vi "returns remaining heater time delay subvi$.vi"(0 "VISA resource name 2":refnum<visa-resource-name>="GPIB0::12::INSTR", 1 "error in (no error) 2":errorcluster) -> (2 "VISA resource name out 2":refnum<visa-resource-name>, 3 "result string":string, 4 "error out 2":errorcluster)   [LabVIEW 2009]
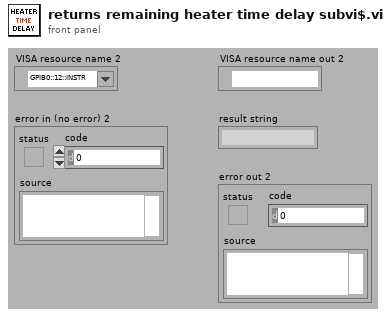
[diagram p1: front panel]
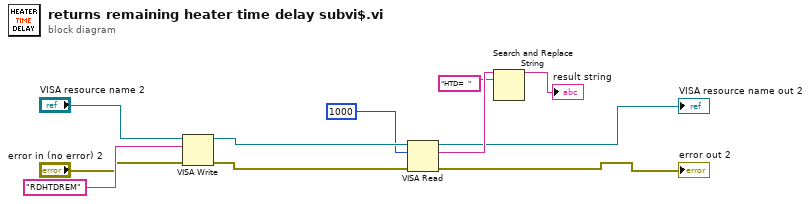
[diagram p0: block diagram]
diagram:
  n1 = VISA Write(VISA resource name="VISA resource name 2", write buffer="RDHTDREM" ("write buffer 2"), error in (no error)="error in (no error) 2") -> (VISA resource name out=w5:refnum<visa-resource-name>, error out=w6:errorcluster)  [unwired: 1 out]
  n2 = VISA Read(VISA resource name=w5, byte count=u32 1000 ("bytes to read (1000) 2"), error in (no error)=w6) -> (VISA resource name out=→"VISA resource name out 2":refnum<visa-resource-name>, read buffer=w11:string, error out=→"error out 2":errorcluster)  [unwired: 1 out]
  n3 = Search and Replace String(input string=w11, search string="HTD=  ") -> (result string=→"result string":string)  [unwired: 6 in, 3 out]
